vi "Remove Bitfile.vi"(8 "error in (no error)":errorcluster, 10 "RIO Device Address":string, 11 "EST Custom Device in":refnum<k24>) -> (0 "error out":errorcluster, 3 "EST Custom Device out":refnum<k24>)   [LabVIEW 2015, in "Engine Simulation Toolkit Scripting API.lvlib"]
uses:
  Engine Simulation Toolkit Scripting API.lvlib
  NationalInstruments.VeriStand.SystemDefinitionAPI
  Shared/Properties.vi
  <vilib>/NI Veristand/Custom Device API/Get Item Property (String Array).vi
  <vilib>/NI Veristand/Custom Device API/Set Item Property (String Array).vi
  Shared/Engine Simulation Toolkit Shared.lvlib
  <vilib>/NI VeriStand/Custom Device API/Custom Device API.lvlib
  System Explorer/Engine Simulation Toolkit System Explorer.lvlib
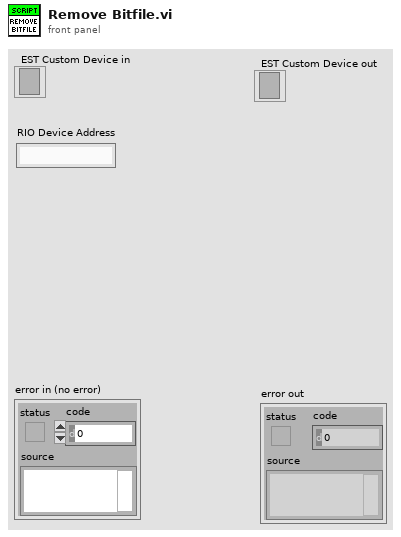
[diagram p1: front panel]
types:
  T1 = typedef "Custom Device API.lvlib/Custom Device Item Ref.ctl" = u64
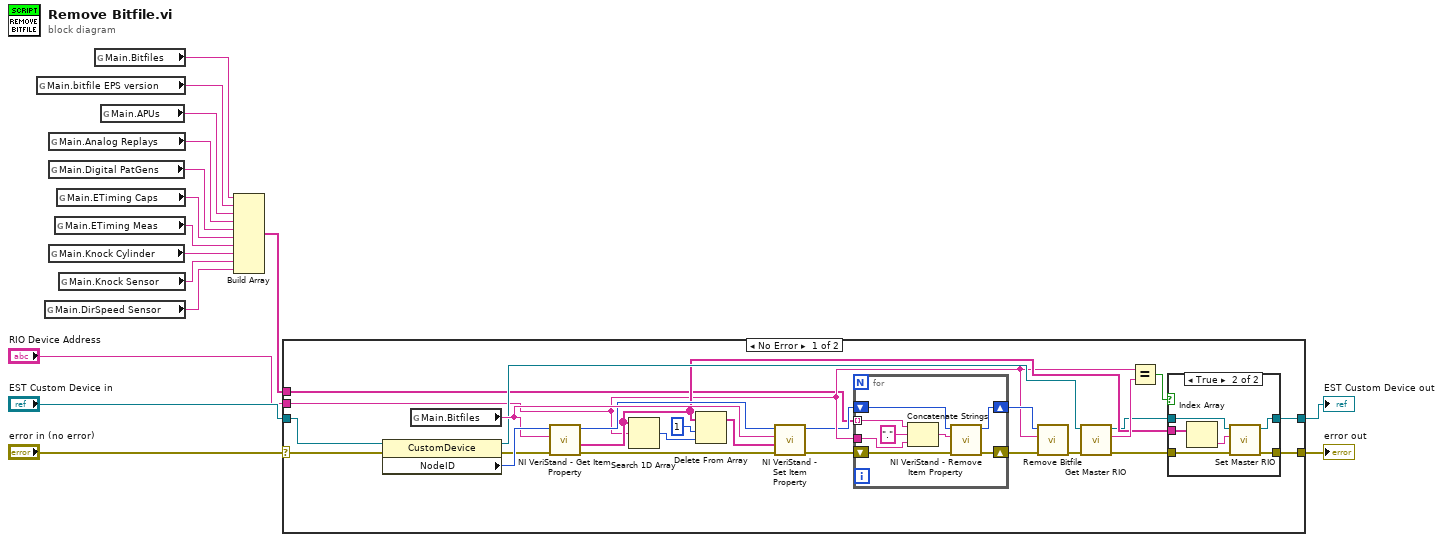
[diagram p0: block diagram]
diagram:
  n1 = global read "Properties.vi" "Main.bitfile EPS version"() -> (w11:string)
  n2 = global read "Properties.vi" "Main.DirSpeed Sensor"() -> (w2:string)
  n3 = global read "Properties.vi" "Main.Analog Replays"() -> (w3:string)
  n4 = global read "Properties.vi" "Main.Digital PatGens"() -> (w4:string)
  n5 = global read "Properties.vi" "Main.Knock Cylinder"() -> (w8:string)
  n6 = global read "Properties.vi" "Main.ETiming Meas"() -> (w6:string)
  n7 = global read "Properties.vi" "Main.ETiming Caps"() -> (w5:string)
  n8 = global read "Properties.vi" "Main.Knock Sensor"() -> (w9:string)
  n9 = global read "Properties.vi" "Main.Bitfiles"() -> (w10:string)
  n10 = global read "Properties.vi" "Main.APUs"() -> (w7:string)
  n11 = Build Array(w10, w11, w7, w3, w4, w5, w6, w8, w9, w2) -> (w1:string[])
  n12 = case shown="No Error" "error in (no error)" {
    selector: "error in (no error)" -> [w40 w59]
    tunnel: [w24 w59] -> w16
    tunnel: "EST Custom Device in" -> [w41 w58]
    tunnel: [w26 w58] -> w13
    tunnel: "RIO Device Address" -> [w19 _]
    tunnel: w1 -> [w17 _]
    frame No Error {
      n13 = property class="CustomDevice"(reference=w41, error in=w40) -> (reference out=w31:refnum<k24>, error out=w32:errorcluster, "NodeID"=w39:u64)
      n14 = global read "Properties.vi" "Main.Bitfiles"() -> (w35:string)
      n15 = call-poly <vilib>:"NI VeriStand - Get Item Property.vi"("error in (no error)"=w32, "Property Name"=w35, "Item Ref in"=w39) -> ("error out"=w33:errorcluster, "Value"=w29:string[], "Item Ref out"=w34:T1)  [unwired: 5 in, 1 out]
      n16 = Search 1D Array(1D array=w29, element=w19) -> (index of element=w38:i32)  [unwired: 1 in]
      n17 = Delete From Array(array=w29, length=1, index=w38) -> (array with subset deleted=w36:string[])  [unwired: 1 out]
      n18 = call-poly <vilib>:"NI VeriStand - Set Item Property.vi"("error in (no error)"=w33, "Value"=w36, "Property Name"=w35, "Item Ref in"=w34) -> ("error out"=w20:errorcluster, "Item Ref out"=w18:T1)  [unwired: 5 in, 1 out]
      n19 = for {
        shift-right: [w48] -> w23
        shift-left: w20 -> [w49]
        tunnel: w17 -> [w44] mode=indexing
        tunnel: w19 -> [w43]
        shift-right: [w45] -> w22
        shift-left: w18 -> [w42]
        n20 = Concatenate Strings(w44, "." ("string"), w43) -> (w46:string)
        n21 = call <vilib>:"NI VeriStand - Remove Item Property.vi"("error in (no error)"=w49, "Property Name"=w46, "Item Ref in"=w42) -> ("error out"=w48:errorcluster, "Item Ref out"=w45:T1)  [unwired: 6 in, 1 out]
      }
      n22 = call "Remove Bitfile.vi"("error in (no error)"=w23, "RIO name"=w19, "Item Ref in"=w22) -> ("error out"=w21:errorcluster)  [unwired: 7 in, 1 out]
      n23 = call "Get Master RIO.vi"("error in (no error)"=w21, "EST Custom Device in"=w31) -> ("error out"=w25:errorcluster, "RIO Device Address"=w30:string, "EST Custom Device out"=w27:refnum<k24>)  [unwired: 7 in]
      n24 = Equal?(x=w19, y=w30) -> (x = y?=w28:bool)
      n25 = case shown="True" w28 {
        tunnel: w29 -> [_ w57]
        tunnel: w27 -> [w51 w55]
        tunnel: [w51 w54] -> w26
        tunnel: w25 -> [w50 w53]
        tunnel: [w50 w52] -> w24
        frame False {
        }
        frame True {
          n26 = Index Array(array=w57) -> (element=w56:string)  [unwired: 1 in]
          n27 = call "Set Master RIO.vi"("error in (no error)"=w53, "RIO Device Address"=w56, "EST Custom Device in"=w55) -> ("error out"=w52:errorcluster, "EST Custom Device out"=w54:refnum<k24>)  [unwired: 7 in]
        }
      }
    }
    frame Error {
    }
  }
  "EST Custom Device out" <- w13
  "error out" <- w16
